vi "Example - Call endpoint.vi"() -> ()   [LabVIEW 2020, in "wamplv.lvlib"]
uses:
  wamplv.lvlib
  WAMP Client/API/TypeDefs/Serialisation.ctl
  0748ca70-c771-45d1-a049-0e3afa802e33.vi
  <vilib>/JDP Science/JSONtext/Variant to JSON Text.vi
  WAMP Client/API/WAMP/JSON/Call JSON.vi
  <vilib>/JDP Science/JSONtext/LVClass Serializer/JSONtext LVClass Serializer.lvclass
  WAMP Client/WAMP Client.lvclass
panel:
  out "Result ArgumentKw Payload":string
  out "Result Arguments Payload":string
  in  "Call Arguments":string[](array[string])
  in  "Endpoint URI":string="test.topic"
  in  "Realm":string="default_realm"
  in  "Router URL":string="ws://localhost:8080/"
  # "Example: call endpoint"
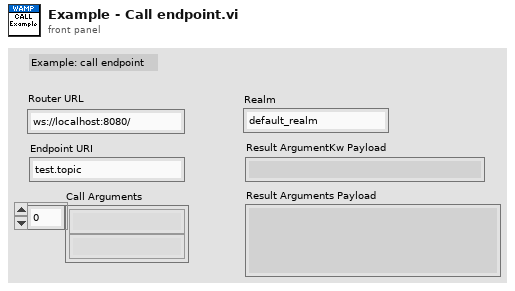
[diagram p1: front panel]
types:
  T1 = typedef "wamplv.lvlib/WAMP Client.lvclass/Serialisation.ctl" = enum16{"JSON", "MessagePack"}
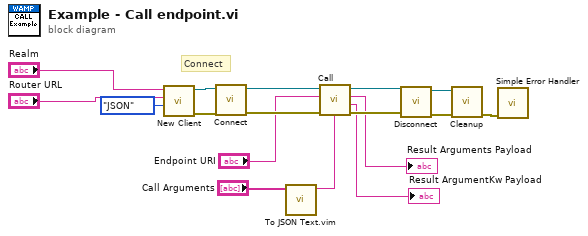
[diagram p0: block diagram]
diagram:
  # "Connect"
  n1 = call "New Client.vi"("Serialisation"=Serialisation."JSON", "Address"="Router URL", "Realm"="Realm") -> ("error out"=w12:errorcluster, "WAMP client out"=w15:refnum<class "WAMP Client.lvclass">)  [unwired: 7 in]
  n2 = call "Connect.vi"("error in"=w12, "WAMP Client in"=w15) -> ("error out"=w7:errorcluster, "WAMP Client out"=w10:refnum<class "WAMP Client.lvclass">)  [unwired: 8 in]
  n3 = call "To JSON Text.vim"("Anything"="Call Arguments") -> ("<JSON>"=w4:string)  [unwired: 9 in, 1 out]
  n4 = call-poly "Call.vi"("Arguments"=w4, "Error in"=w7, "Topic URI"="Endpoint URI", "WAMP Client in"=w10) -> ("Error out"=w8:errorcluster, "ArgumentKw Payload"=→"Result ArgumentKw Payload":string, "Arguments Payload"=→"Result Arguments Payload":string, "WAMP Client out"=w9:refnum<class "WAMP Client.lvclass">)  [unwired: 3 in, 1 out]
  n5 = call-dynamic "Disconnect.vi"("error in"=w8, "WAMP Client in"=w9) -> ("error out"=w11:errorcluster, "WAMP Client out"=w14:refnum<class "WAMP Client.lvclass">)  [unwired: 8 in]
  n6 = call-dynamic "Cleanup.vi"("error in"=w11, "WAMP Client in"=w14) -> ("error out"=w13:errorcluster)  [unwired: 8 in, 1 out]
  n7 = call <vilib>:"Simple Error Handler.vi"("error in (no error)"=w13) -> ()  [unwired: 4 in, 5 out]
